vi "NATS HPUB.vi"(5 "headers":string, 6 "timeout ms (conn default)":i32=-2, 7 "reply-to":string, 8 "error in":errorcluster, 9 "payload":string, 10 "subject":string, 11 "nats connection in":T1={"connection ID"=refnum, "server INFO"="", "timeout ms"=5000, "verbose?"=FALSE, "server headers?"=FALSE, "client headers?"=FALSE}) -> (0 "error out":errorcluster, 3 "dup nats connection":T1={"connection ID"=refnum, "server INFO"="", "timeout ms"=5000, "verbose?"=FALSE, "server headers?"=FALSE, "client headers?"=FALSE})   [LabVIEW 2013, in "NATS Core.lvlib"]
doc: "Publishes a message with headers to the NATS server."
uses:
  NATS Core.lvlib
  Controls/nats connection.ctl
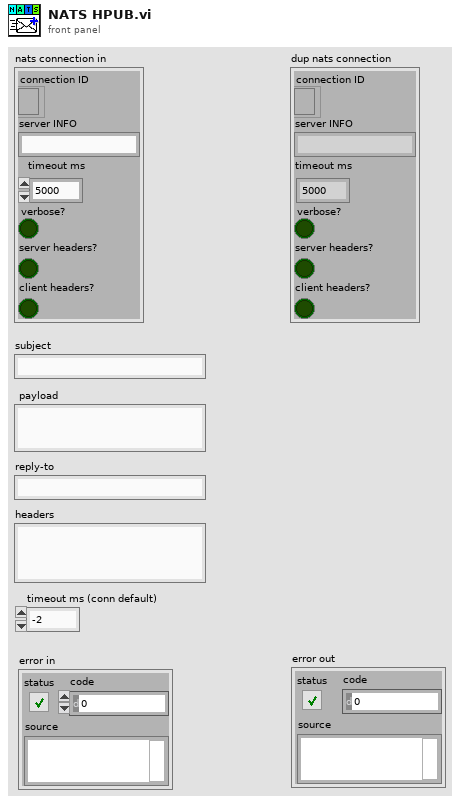
[diagram p1: front panel]
types:
  T1 = typedef "NATS Core.lvlib/nats connection.ctl" = cluster{"connection ID":refnum<k5>, "server INFO":string, "timeout ms":i32, "verbose?":bool, "server headers?":bool, "client headers?":bool}
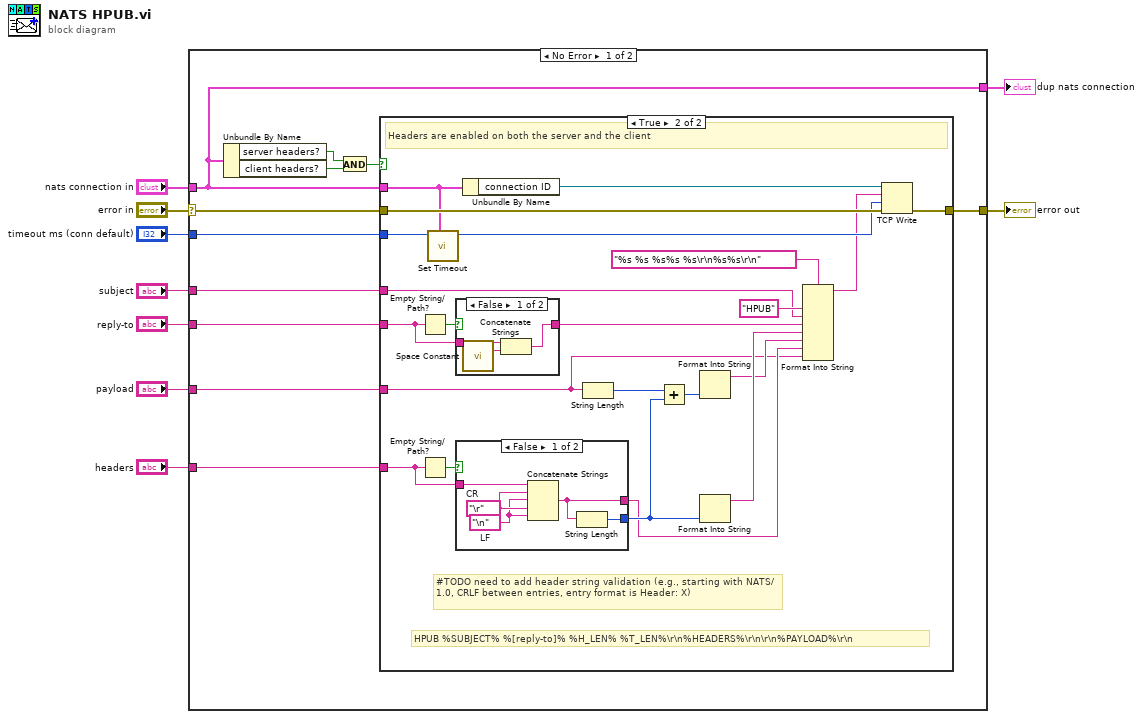
[diagram p0: block diagram]
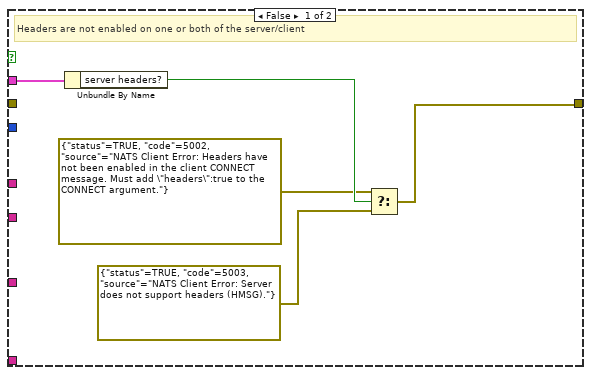
[diagram p2: hidden frame]
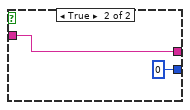
[diagram p3: hidden frame]
diagram:
  n1 = case shown="No Error" "error in" {
    selector: "error in" -> [w20 w60]
    tunnel: "nats connection in" -> [w13 w59]
    tunnel: "timeout ms (conn default)" -> [w18 _]
    tunnel: [w19 w60] -> w6
    tunnel: "subject" -> [w15 _]
    tunnel: "payload" -> [w14 _]
    tunnel: [w13 w59] -> w3
    tunnel: "reply-to" -> [w17 _]
    tunnel: "headers" -> [w16 _]
    frame No Error {
      n2 = Unbundle By Name(w13) -> ("server headers?"=w11:bool, "client headers?"=w12:bool)
      n3 = And(x=w11, y=w12) -> (x .and. y?=w10:bool)
      n4 = case shown="True" w10 {
        tunnel: w20 -> [_ w47]
        tunnel: [w21 w45] -> w19
        tunnel: w13 -> [w25 w44]
        tunnel: w18 -> [_ w43]
        tunnel: w17 -> [_ w40]
        tunnel: w16 -> [_ w38]
        tunnel: w15 -> [_ w32]
        tunnel: w14 -> [_ w27]
        frame False {
          # "Headers are not enabled on one or both of the server/client"
          n5 = Unbundle By Name(w25) -> ("server headers?"=w24:bool)
          n6 = Select(t=errorcluster {"status"=TRUE, "code"=5002, "source"="NATS Client Error: Headers have not been enabled in the client CONNECT message. Must add \"headers\":true to the CONNECT argument."} ("error constant"), s=w24, f=errorcluster {"status"=TRUE, "code"=5003, "source"="NATS Client Error: Server does not support headers (HMSG)."} ("error constant")) -> (s? t:f=w21:errorcluster)
        }
        frame True {
          # "#TODO need to add header string validation (e.g., starting with NATS/1.0, CRLF between entries, entry format is Header: X)"
          # "HPUB %SUBJECT% %[reply-to]% %H_LEN% %T_LEN%\\r\\n%HEADERS%\\r\\n\\r\\n%PAYLOAD%\\r\\n"
          # "Headers are enabled on both the server and the client"
          n7 = Empty String/Path?(string/path=w40) -> (empty?=w41:bool)
          n8 = Empty String/Path?(string/path=w38) -> (empty?=w39:bool)
          n9 = call "Set Timeout.vi"("nats connection in"=w44, "timeout ms in"=w43) -> ("timeout ms out"=w42:i32)  [unwired: 9 in]
          n10 = case shown="False" w41 {
            tunnel: w40 -> [w57 w58]
            tunnel: [w55 w58] -> w31
            frame False {
              n11 = call <vilib>:"Space Constant.vi"() -> ("String"=w56:string)
              n12 = Concatenate Strings(w57, w56) -> (w55:string)
            }
            frame True {
            }
          }
          n13 = case shown="False" w39 {
            tunnel: w38 -> [w52 w54]
            tunnel: [w49 w54] -> w28
            tunnel: [w48 0] -> w35
            frame False {
              w50 = "\n"  # LF
              w51 = "\r"  # CR
              n14 = Concatenate Strings(w52, w51, w50, w51, w50) -> (w49:string)
              n15 = String Length(string=w49) -> (length=w48:i32)
            }
            frame True {
            }
          }
          n16 = Unbundle By Name(w44) -> ("connection ID"=w46:refnum<k5>)
          n17 = String Length(string=w27) -> (length=w37:i32)
          n18 = Add(x=w37, y=w35) -> (x+y=w36:i32)
          n19 = Format Into String(w36) -> (resulting string=w29:string)  [unwired: 3 in, 1 out]
          n20 = Format Into String(w35) -> (resulting string=w30:string)  [unwired: 3 in, 1 out]
          n21 = Format Into String(format string="%s %s %s%s %s\r\n%s%s\r\n", "HPUB" ("input 1"), w32, w31, w30, w29, w28, w27) -> (resulting string=w26:string)  [unwired: 2 in, 1 out]
          n22 = TCP Write(connection ID=w46, data in=w26, error in (no error)=w47, 9:w42) -> (error out=w45:errorcluster)  [unwired: 2 out]
        }
      }
    }
    frame Error {
    }
  }
  "error out" <- w6
  "dup nats connection" <- w3
